vi "Translation2d_Interpolate.vi"(9 "T":dbl, 10 "other Translation":T1 {"Y" format="%14.3f"; "X" format="%14.3f"}, 11 "In Translation":T1 {"Y" format="%14.3f"; "X" format="%14.3f"}) -> (3 "Interpolated Translation":T1 {"Y" format="%14.3f"; "X" format="%14.3f"})   [LabVIEW 2019, in "Trajectory_Library.lvlib"]
doc: "Inerpolate between this and an End Value translation\n \n\nParameters:\n - IN Translation - This translation data structure\n - EndValue Translation - The translation data structure\n\nReturns\n - Interpolated Translation - The interpolated translation."
uses:
  Trajectory_Library.lvlib
  TRANSLATION2D.ctl
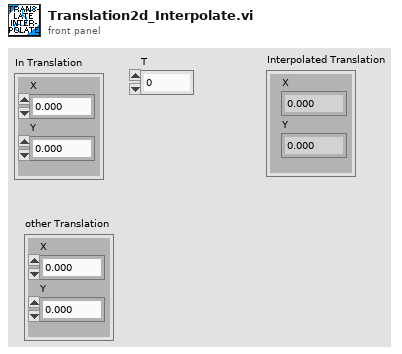
[diagram p1: front panel]
types:
  T1 = typedef "Trajectory_Library.lvlib/TRANSLATION2D.ctl" = cluster{"X":dbl, "Y":dbl}
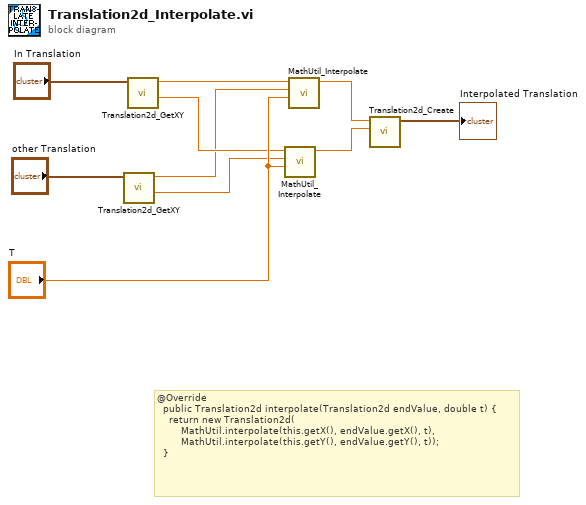
[diagram p0: block diagram]
diagram:
  # "@Override\n  public Translation2d interpolate(Translation2d endValue, double t) {\n    return new Translation2d(\n        MathUtil.interpolate(this.getX(), endValue.getX(), t),\n        MathUtil.interpolate(this.getY(), endValue.getY(), t));\n  }"
  n1 = call "Translation2d_GetXY.vi"("In Translation"="other Translation") -> ("Y"=w2:dbl, "X"=w3:dbl)  [unwired: 9 in]
  n2 = call "Translation2d_GetXY.vi"("In Translation"="In Translation") -> ("Y"=w5:dbl, "X"=w6:dbl)  [unwired: 9 in]
  n3 = call "MathUtil_Interpolate.vi"("T"="T", "EndValue"=w2, "StartValue"=w5) -> ("InterpolatedValue"=w7:dbl)  [unwired: 8 in]
  n4 = call "MathUtil_Interpolate.vi"("T"="T", "EndValue"=w3, "StartValue"=w6) -> ("InterpolatedValue"=w8:dbl)  [unwired: 8 in]
  n5 = call "Translation2d_Create.vi"("Y"=w7, "X"=w8) -> ("TRANSLATION"=→"Interpolated Translation":T1)  [unwired: 9 in]
